vi "LockinDAQ.Read AI and Write AO.vi"(8 "error in (no error)":errorcluster, 10 "AO []":waveform(dbl)[](array[waveform]), 11 "LockinDAQ":refnum<class "LockinDAQ.lvclass">) -> (0 "error out":errorcluster, 2 "AI []":waveform(dbl)[](array[waveform]), 3 "LockinDAQ out":refnum<class "LockinDAQ.lvclass">)   [LabVIEW 2016, in "LockinDAQ.lvclass"]
uses:
  LockinDAQ.lvclass
panel:
  out "AO":u32
  out "AI":u32
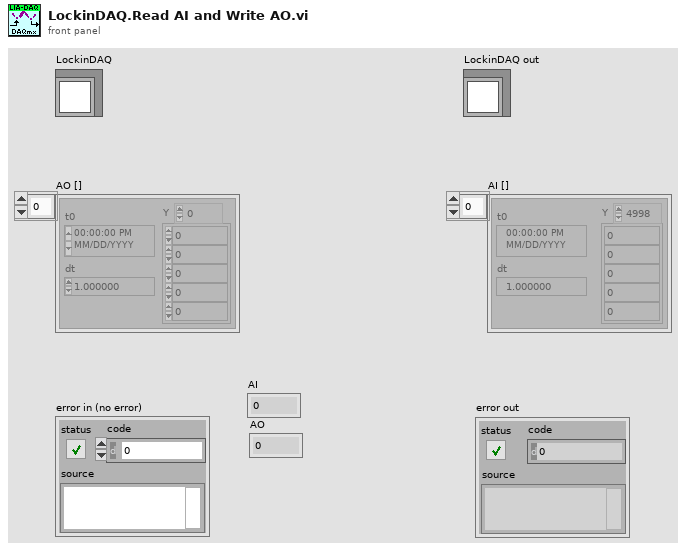
[diagram p1: front panel]
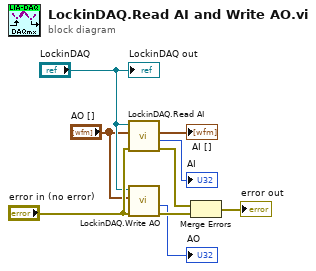
[diagram p0: block diagram]
diagram:
  n1 = call "LockinDAQ.Read AI.vi"("error in (no error)"="error in (no error)", "AO []"="AO []", "LockinDAQ"="LockinDAQ") -> ("error out"=w5:errorcluster, "AI"=→"AI":u32, "AI []"=→"AI []":waveform(dbl)[])  [unwired: 5 in, 1 out]
  n2 = call "LockinDAQ.Write AO.vi"("error in (no error)"="error in (no error)", "AO []"="AO []", "LockinDAQ"="LockinDAQ") -> ("error out"=w7:errorcluster, "AO"=→"AO":u32)  [unwired: 6 in, 1 out]
  n3 = Merge Errors(w5, w7) -> (→"error out":errorcluster)
  "LockinDAQ out" <- "LockinDAQ"
